vi "Create PWM Input Channel.vi"(6 "index":i32, 7 "measurement type":T1, 8 "error in":errorcluster, 9 "default value":dbl, 10 "name":string, 11 "PWM input channel in":refnum<class "PWM Input Channel.lvclass">) -> (0 "error out":errorcluster, 3 "PWM input channel out":refnum<class "PWM Input Channel.lvclass">)   [LabVIEW 2020, in "Scan Engine Scripting.lvlib" / "PWM Input Channel.lvclass"]
uses:
  PWM Input Channel.lvclass
  Measurement Type.ctl
  Channel/Type.ctl
  Channel/Channel.lvclass
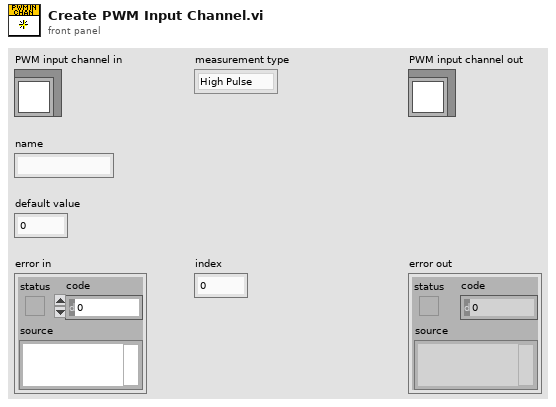
[diagram p1: front panel]
types:
  T1 = typedef "Scan Engine Scripting.lvlib/PWM Input Channel.lvclass/Measurement Type.ctl" = enum16{"High Pulse", "Low Pulse", "Most Recent"}
  T2 = typedef "Scan Engine Scripting.lvlib/Channel.lvclass/Type.ctl" = enum16{"Input", "Output"}
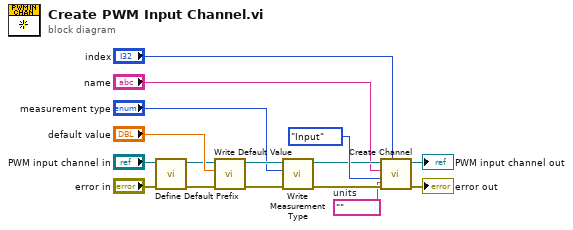
[diagram p0: block diagram]
diagram:
  w1 = ""  # units
  n1 = call-dynamic "Define Default Prefix.vi"("error in"="error in", "PWM input channel in"="PWM input channel in") -> ("error out"=w2:errorcluster, "PWM input channel out"=w4:refnum<class "PWM Input Channel.lvclass">)  [unwired: 8 in]
  n2 = call-dynamic "Write Default Value.vi"("error in"=w2, "default value"="default value", "PWM channel in"=w4) -> ("error out"=w13:errorcluster, "PWM channel out"=w14:refnum<class "PWM Input Channel.lvclass">)  [unwired: 7 in]
  n3 = call-dynamic "Write Measurement Type.vi"("error in"=w13, "measurement type"="measurement type", "PWM input channel in"=w14) -> ("error out"=w11:errorcluster, "PWM input channel out"=w12:refnum<class "PWM Input Channel.lvclass">)  [unwired: 7 in]
  n4 = call-dynamic "Create Channel.vi"("units"=w1, "index"="index", "error in"=w11, "type"=Type."Input", "name"="name", "channel in"=w12) -> ("error out"=→"error out":errorcluster, "channel out"=→"PWM input channel out":refnum<class "PWM Input Channel.lvclass">)  [unwired: 4 in]
